vi "apply error handling configuration.vi"(8 "error in":errorcluster, 10 "configuration in":refnum<class "control module configuration.lvclass">, 11 "fixed channel runtime in":refnum<class "control module runtime.lvclass">) -> (0 "error out":errorcluster, 3 "fixed channel runtime out":refnum<class "control module runtime.lvclass">)   [LabVIEW 2013, in "control module runtime.lvclass"]
uses:
  control module runtime.lvclass
  configuration/control module configuration.lvclass
  configuration/control module configuration.lvclass/control module configuration.ctl
  control module runtime.lvclass/control module runtime.ctl
  configuration/Read error classifications.vi
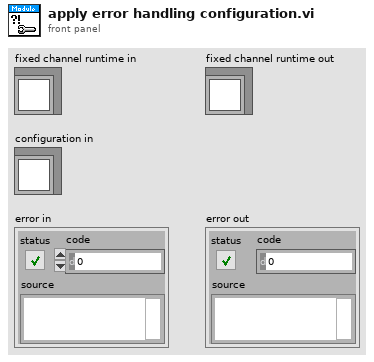
[diagram p1: front panel]
types:
  T1 = typedef "control module configuration.lvclass/error classification.ctl" = cluster{"code":i32, "error classification":T2}
  T2 = typedef "TBM module execution interface.lvclass/error classification.ctl" = enum16{"unknown", "none", "trivial", "recoverable", "critical"}
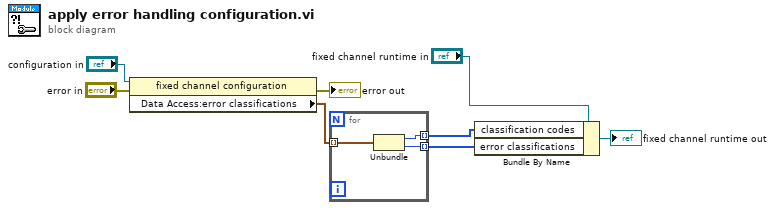
[diagram p0: block diagram]
diagram:
  n1 = property class="fixed channel configuration"(reference="configuration in", error in="error in") -> (error out=→"error out":errorcluster, "Data Access:error classifications"=w3:T1[])  [unwired: 1 out]
  n2 = for {
    tunnel: w3 -> [w11] mode=indexing
    tunnel: [w10] -> w2 mode=indexing
    tunnel: [w9] -> w1 mode=indexing
    n3 = Unbundle(w11) -> ("code"=w10:i32, "error classification"=w9:T2)
  }
  n4 = Bundle By Name(cluster="fixed channel runtime in", "classification codes"=w2, "error classifications"=w1) -> (→"fixed channel runtime out":refnum<class "control module runtime.lvclass">)
